vi "AutoFollowTrajectory.vi"(8 "error in (no error)":errorcluster, 9 "TimeOut (s)":dbl, 11 "Trajectory":T1 {"States"."POSE"."ROTATION"."SIN" format="%13.4f"; "States"."POSE"."ROTATION"."COS" format="%13.4f"; "States"."POSE"."ROTATION"."VALUE" format="%13.4f"; "States"."POSE"."TRANSLATION"."Y" format="%14.3f"; "States"."POSE"."TRANSLATION"."X" format="%14.3f"; "TotalTImeSecs" format="%20.3f"}) -> (0 "error out":errorcluster)   [LabVIEW 2020]
doc: "Wrapper class for drive straight"
uses:
  <vilib>/Rock Robotics/WPI/ThirdParty/JAS_Junk/TrajLib/Trajectory_Library.lvlib
  <vilib>/Rock Robotics/WPI/ThirdParty/JAS_Junk/TrajLib/TypeDef/TRANSLATION2D.ctl
  <vilib>/Rock Robotics/WPI/ThirdParty/JAS_Junk/TrajLib/TypeDef/ROTATION2D.ctl
  <vilib>/Rock Robotics/WPI/ThirdParty/JAS_Junk/TrajLib/TypeDef/POSE2D.ctl
  <vilib>/Rock Robotics/WPI/ThirdParty/JAS_Junk/TrajLib/TypeDef/TRAJ_STATE.ctl
  <vilib>/Rock Robotics/WPI/ThirdParty/JAS_Junk/TrajLib/TypeDef/TRAJECTORY.ctl
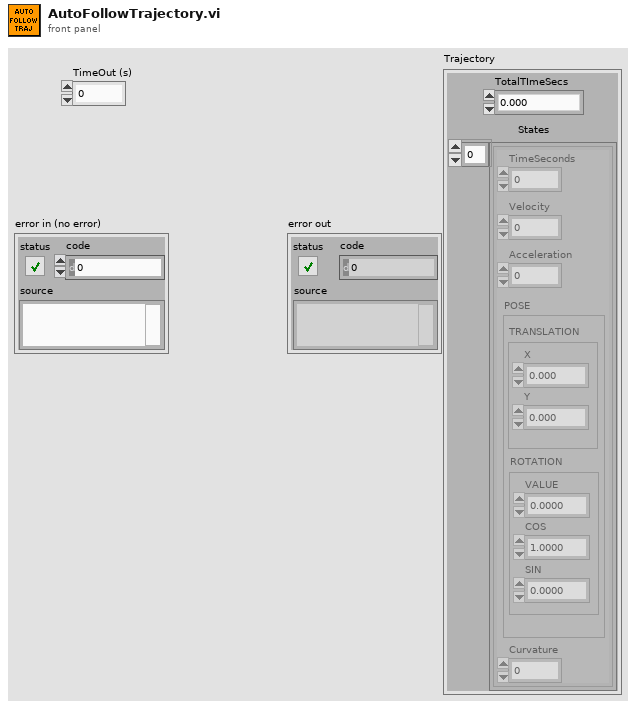
[diagram p1: front panel]
types:
  T1 = typedef "Trajectory_Library.lvlib/TRAJECTORY.ctl" = cluster{"TotalTImeSecs":dbl, "States":T2[]}
  T2 = typedef "Trajectory_Library.lvlib/TRAJ_STATE.ctl" = cluster{"TimeSeconds":dbl, "Velocity":dbl, "Acceleration":dbl, "POSE":T3, "Curvature":dbl}
  T3 = typedef "Trajectory_Library.lvlib/POSE2D.ctl" = cluster{"TRANSLATION":T4, "ROTATION":T5}
  T4 = typedef "Trajectory_Library.lvlib/TRANSLATION2D.ctl" = cluster{"X":dbl, "Y":dbl}
  T5 = typedef "Trajectory_Library.lvlib/ROTATION2D.ctl" = cluster{"VALUE":dbl, "COS":dbl, "SIN":dbl}
  T6 = typedef "Trajectory_Library.lvlib/TIMER.ctl" = cluster{"StartTime":dbl, "Accumulated TIme":dbl, "Running":bool, "semaphore":T7}
  T7 = typedef "Semaphore RefNum" = refnum<k1>
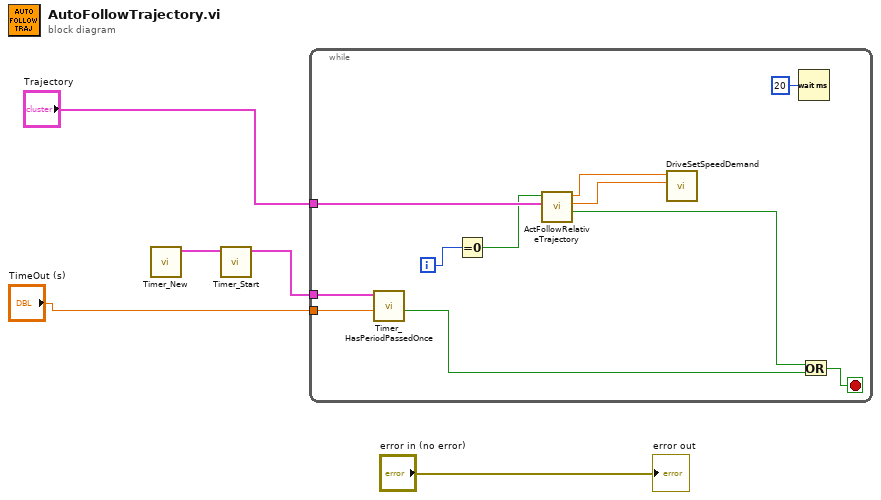
[diagram p0: block diagram]
diagram:
  n1 = call <vilib>:"Timer_New.vi"() -> ("TIMER"=w4:T6)  [unwired: 11 in]
  n2 = call <vilib>:"Timer_Start.vi"("in Timer"=w4) -> ("out Timer"=w3:T6)  [unwired: 10 in]
  n3 = while {
    tunnel: w3 -> [w15]
    tunnel: "TimeOut (s)" -> [w14]
    tunnel: "Trajectory" -> [w10]
    i -> [w16]
    stop <- w12 stop-if-true
    n4 = call <vilib>:"Timer_HasPeriodPassedOnce.vi"("Period"=w14, "in Timer"=w15) -> ("Expired"=w13:bool)  [unwired: 7 in, 2 out]
    n5 = Equal To 0?(x=w16) -> (x = 0?=w6:bool)
    n6 = call "ActFollowRelativeTrajectory.vi"("Trajectory"=w10, "FirstTime"=w6) -> ("Done"=w9:bool, "RightSpeed"=w8:dbl, "LeftSpeed"=w7:dbl)  [unwired: 7 in]
    n7 = call "DriveSetSpeedDemand.vi"("YSpeedDemand (ft/s)"=w8, "XSpeedDemand (ft/s)"=w7) -> ()  [unwired: 10 in]
    n8 = Wait (ms)(milliseconds to wait=u32 20) -> ()  [unwired: 1 out]
    n9 = Or(x=w9, y=w13) -> (x .or. y?=w12:bool)
  }
  "error out" <- "error in (no error)"
